vi "Change Frame Names.vi"(8 "error in (no error)":errorcluster, 11 "case structure in":refnum<vi>) -> (0 "error out":errorcluster, 3 "case structure out":refnum<vi>)   [LabVIEW 2017]
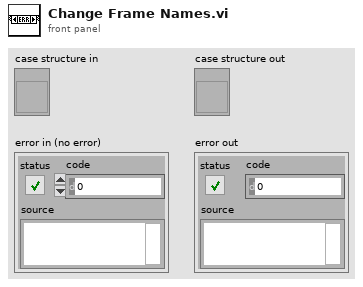
[diagram p1: front panel]
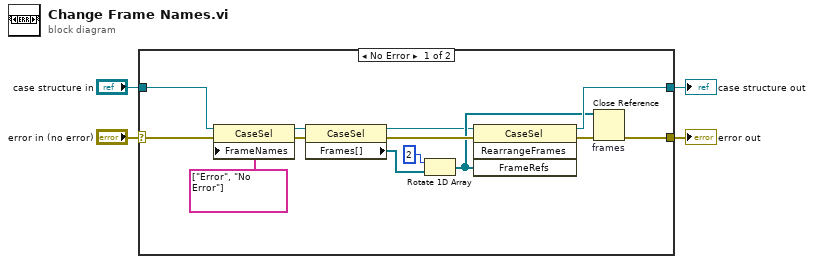
[diagram p0: block diagram]
diagram:
  n1 = case shown="No Error" "error in (no error)" {
    selector: "error in (no error)" -> [w8 w19]
    tunnel: [w17 w18] -> w4
    tunnel: [w7 w19] -> w3
    tunnel: "case structure in" -> [w15 w18]
    frame No Error {
      n2 = property class="CaseSel"(reference=w15, error in=w8, "FrameNames"=string[] ["Error", "No Error"] ("Frame Names")) -> (reference out=w11:refnum<vi>, error out=w9:errorcluster)
      n3 = property class="CaseSel"(reference=w11, error in=w9) -> (reference out=w5:refnum<vi>, error out=w10:errorcluster, "Frames[]"=w12:refnum<vi>[])
      n4 = Rotate 1D Array(1:w12, 2:2 ("n")) -> (0:w6:refnum<vi>[])
      n5 = invoke class="CaseSel" method="RearrangeFrames"(reference=w5, error in=w10, "FrameRefs"=w6) -> (reference out=w17:refnum<vi>, error out=w16:errorcluster)  [unwired: 1 in, 2 out]
      n6 = Close Reference "frames"(reference=w6, error in (no error)=w16) -> (error out=w7:errorcluster)
    }
    frame Error {
    }
  }
  "case structure out" <- w4
  "error out" <- w3
